vi "Day01-02.vi"() -> ()   [LabVIEW 2021]
uses:
  2b6feea8-4815-4cd8-ae99-f2c110e22a6b.vi
  <vilib>/Comparison/Equal/Equal Functor/Equal Functor.lvclass
panel:
  out "마지막 값":i32
  out "조건적":i32[](array[numeric])
  out "인덱스 하기":i32[](array[numeric])
  out "배열":dbl[](array[numeric])
  out "숫자형 3":dbl
  out "숫자형 2":i32
  in  "STOP 2":bool
  out "x+y 4":dbl
  in  "x 2":dbl
  in  "y 2":dbl
  out "x+y 3":dbl
  in  "y":dbl
  in  "x":dbl
  in  "STOP":bool
  out "숫자형":i32
  out "증가 값":dbl[](array[numeric])
  in  "인덱스":dbl
  in  "원래 값":dbl[](array[numeric])
  out "출력 클러스터 2":cluster{"금액":dbl, "버튼":bool, "상태창":string}
  out "출력 클러스터":cluster{"금액":dbl, "버튼":bool, "상태창":string}
  out "클러스터어어 5":cluster{"숫자랑 배열":dbl[], "버튼":bool, "상태창":string}
  in  "클러스터어어 4":cluster{"숫자랑 배열":dbl[], "버튼":bool, "상태창":string}
  in  "클러스터어어 3":cluster{"금액":dbl, "버튼":bool, "상태창":string}
  in  "클러스터어어 2":cluster{"금액":dbl, "버튼":bool, "상태창":string}
  out "상태창":string
  out "버튼":bool
  out "금액":dbl
  in  "클러스터어어":cluster{"금액":dbl, "버튼":bool, "상태창":string}
  out "연결된 문자열":string
  out "길이":i32[](array[numeric])
  out "x .and. y? 2":bool[](array[boolean])
  out "x .and. y?":bool[](array[boolean])
  out "x+y 2":i32[](array[numeric])
  out "x+y":i32[](array[numeric])
  out "index of element":i32 caption="원소의 인덱스"
  out "추가된 배열 5":dbl[](array[numeric])
  out "추가된 배열 4":dbl[][](array[numeric])
  out "추가된 배열 3":dbl[](array[numeric])
  out "추가된 배열 2":dbl[](array[numeric])
  out "추가된 배열":dbl[](array[numeric])
  # "숫자형 함수의 다형성"
  # "불리언 함수의 다형성"
  # "문자형 함수의 다형성"
  # "문자형 함수의 다형성 2"
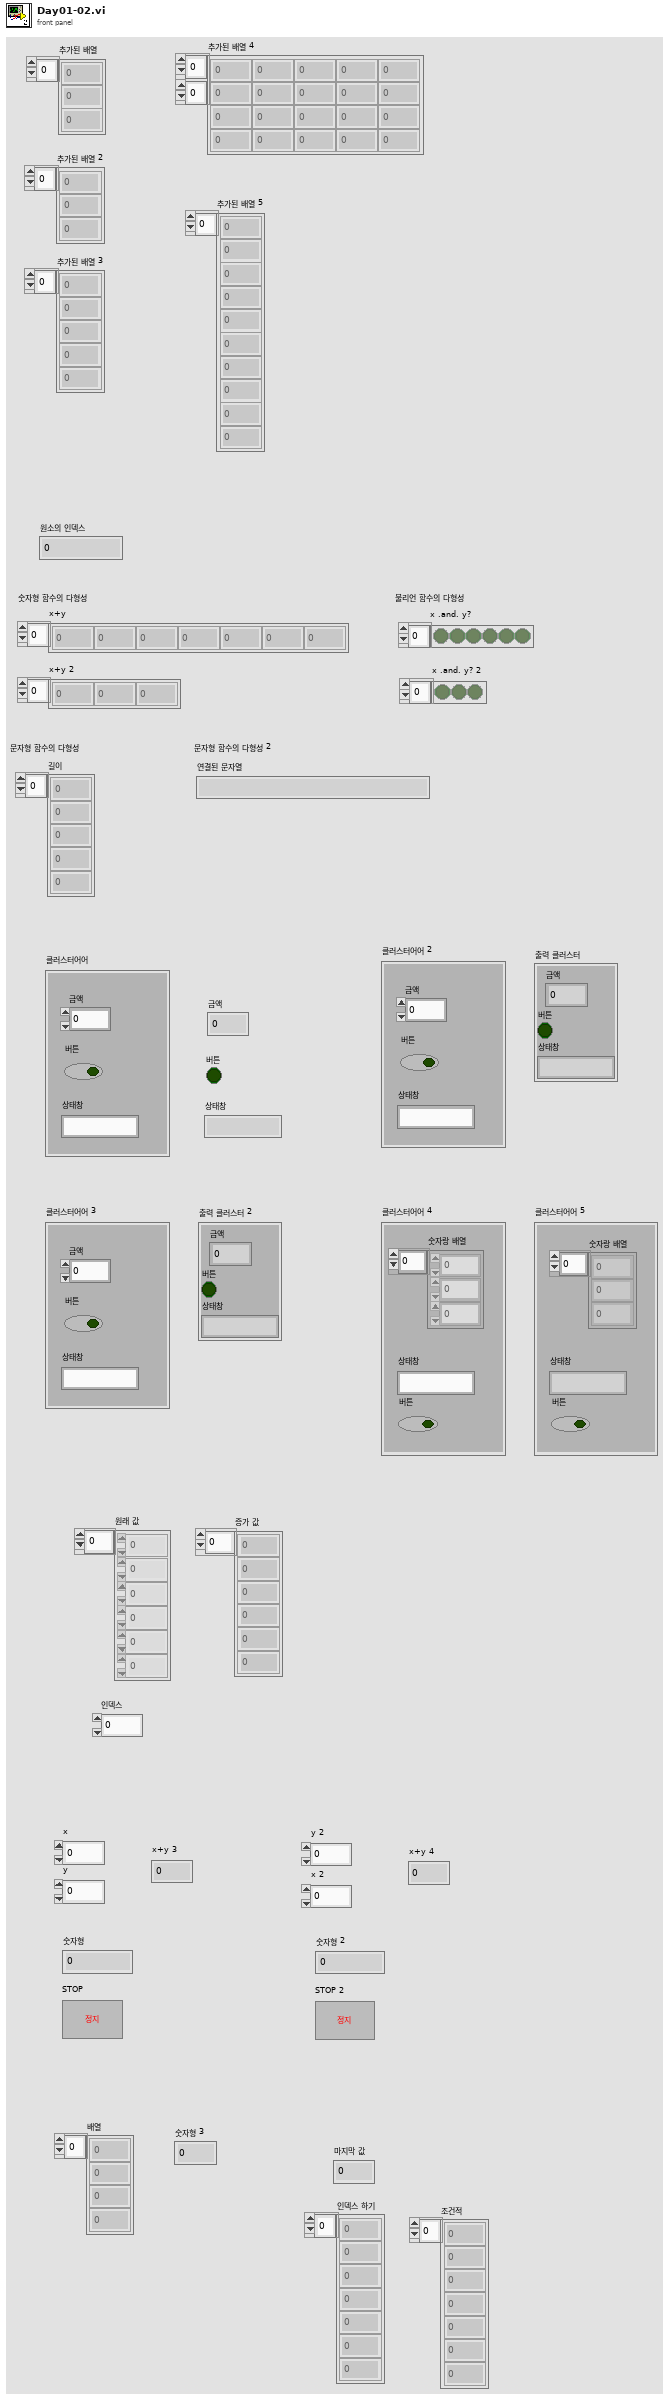
[diagram p1: front panel]
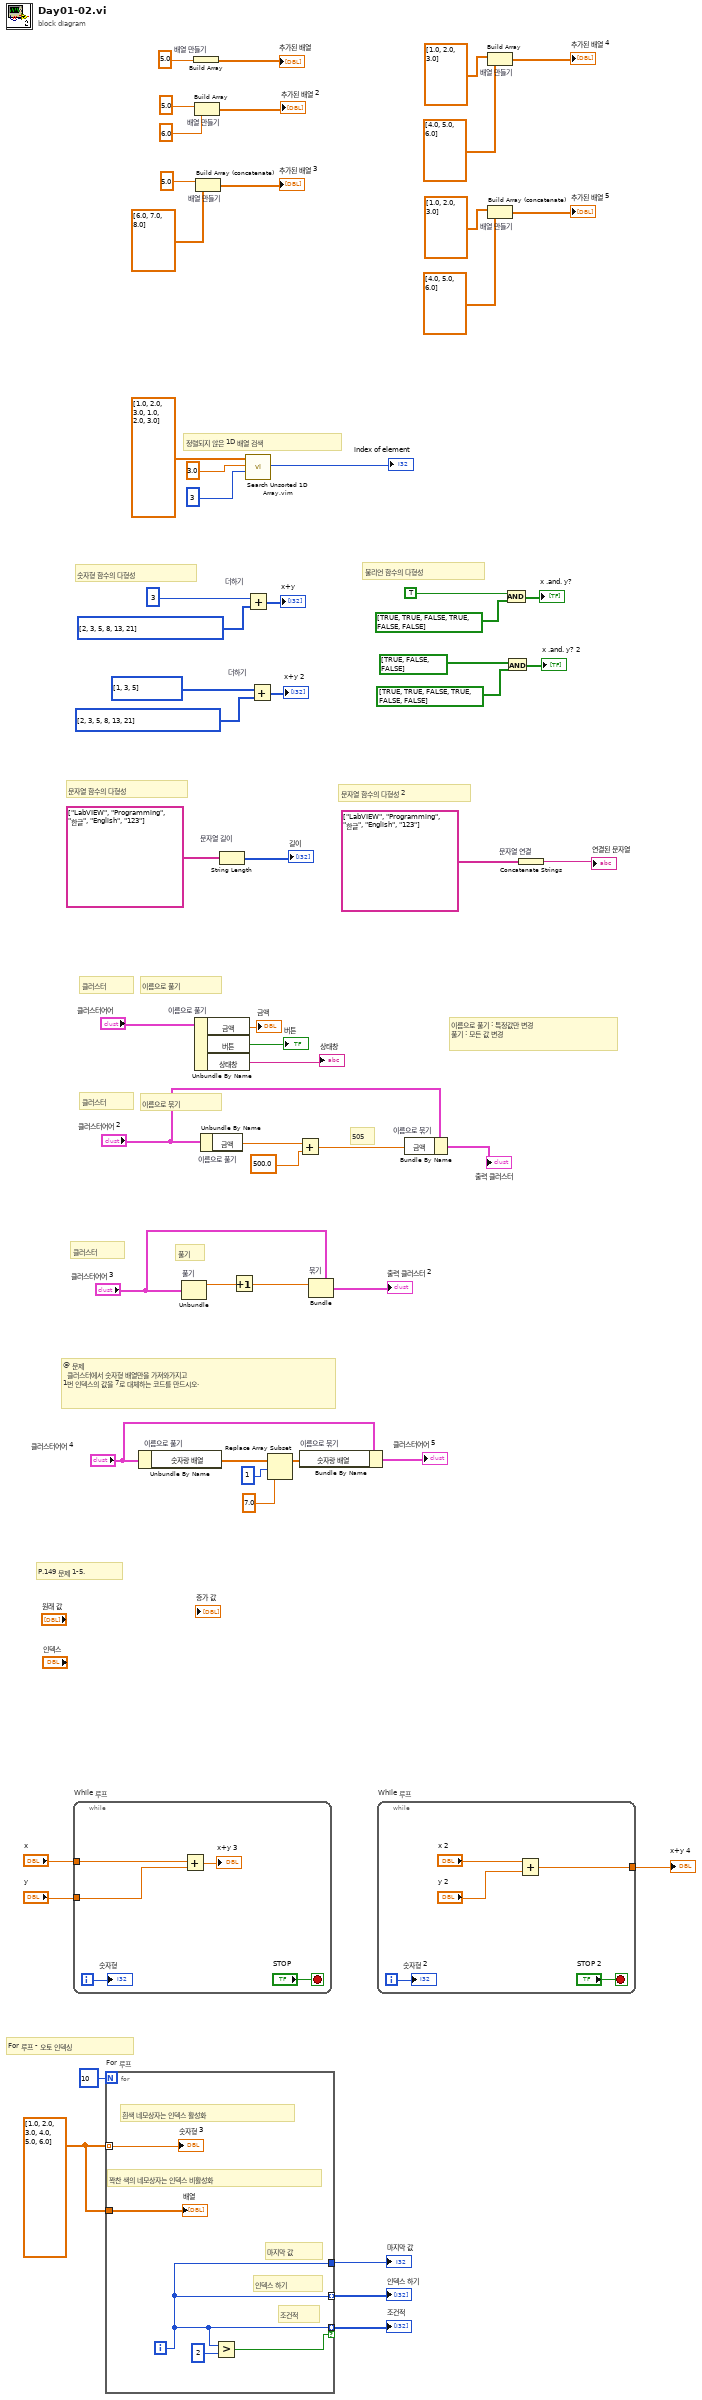
[diagram p0: block diagram]
diagram:
  w4 = dbl[] [1.0, 2.0, 3.0, 4.0, 5.0, 6.0]
  # "For 루프 - 오토 인덱싱"
  # "P.149 문제 1-5."
  # "이름으로 묶기"
  # "505"
  # "@ 문제\n  클러스터에서 숫자형 배열만을 가져와가지고\n1번 인덱스의 값을 7로 대체하는 코드를 만드시오."
  # "클러스터"
  # "이름으로 풀기 : 특정값만 변경\n풀기 : 모든 값 변경"
  # "풀기"
  # "이름으로 풀기"
  # "클러스터"
  # "클러스터"
  # "문자열 함수의 다형성 2"
  # "문자열 함수의 다형성"
  # "불리언 함수의 다형성"
  # "숫자형 함수의 다형성"
  # "정렬되지 않은 1D 배열 검색"
  n1 = while "While 루프" {
    tunnel: "x" -> [w64]
    tunnel: "y" -> [w63]
    i -> [w66]
    stop <- "STOP" stop-if-true
    n2 = Add(x=w64, y=w63) -> (x+y=→"x+y 3":dbl)
    "숫자형" <- w66
  }
  n3 = for "For 루프" {
    N: 10 -> [_]
    tunnel: w4 -> [w71] mode=indexing
    tunnel: w4 -> [w70]
    tunnel: [w69] -> w1
    tunnel: [w69] -> w3 mode=indexing
    tunnel: [w69] -> w2 mode=indexing if=w67
    i -> [w69]
    # "조건적"
    # "인덱스 하기"
    # "마지막 값"
    # "꽉찬 색의 네모상자는 인덱스 비활성화"
    # "흰색 네모상자는 인덱스 활성화"
    n4 = Greater?(x=w69, y=2) -> (0:w67:bool)
    "숫자형 3" <- w71
    "배열" <- w70
  }
  "인덱스 하기" <- w3
  "조건적" <- w2
  "마지막 값" <- w1
  n5 = Unbundle By Name "이름으로 풀기"("클러스터어어 4") -> ("숫자랑 배열"=w18:dbl[])
  n6 = Unbundle "풀기"("클러스터어어 3") -> ("금액"=w23:dbl)  [unwired: 2 out]
  n7 = Build Array "배열 만들기"(5.0 ("원소")) -> (→"추가된 배열":dbl[])
  n8 = Build Array "배열 만들기"(5.0 ("원소"), 6.0 ("원소")) -> (→"추가된 배열 2":dbl[])
  n9 = Unbundle By Name "이름으로 풀기"("클러스터어어") -> ("금액"=→"금액":dbl, "버튼"=→"버튼":bool, "상태창"=→"상태창":string)
  n10 = Build Array (concatenate) "배열 만들기"(5.0 ("원소"), dbl[] [6.0, 7.0, 8.0] ("원소")) -> (→"추가된 배열 3":dbl[])
  n11 = Unbundle By Name "이름으로 풀기"("클러스터어어 2") -> ("금액"=w21:dbl)
  n12 = String Length "문자열 길이"(string=string[] ["LabVIEW", "Programming", "한글", "English", "123"]) -> (length=→"길이":i32[])
  n13 = Increment(x=w23) -> (x+1=w12:dbl)
  n14 = call "Search Unsorted 1D Array.vim"("start index (0)"=3, "element"=3.0, "unsorted 1D array"=dbl[] [1.0, 2.0, 3.0, 1.0, 2.0, 3.0]) -> ("index of element"=→"index of element":i32)  [unwired: 8 in]
  n15 = Add "더하기"(x=3, y=i32[] [2, 3, 5, 8, 13, 21]) -> (x+y=→"x+y":i32[])
  n16 = Add "더하기"(x=i32[] [1, 3, 5], y=i32[] [2, 3, 5, 8, 13, 21]) -> (x+y=→"x+y 2":i32[])
  n17 = Replace Array Subset(array=w18, new element=7.0 ("새 원소/부분배열"), index=1 ("인덱스")) -> (w15:dbl[])
  n18 = Add(x=w21, y=500.0) -> (x+y=w22:dbl)
  n19 = Bundle By Name "이름으로 묶기"(cluster="클러스터어어 4", "숫자랑 배열"=w15) -> (→"클러스터어어 5":cluster{"숫자랑 배열":dbl[], "버튼":bool, "상태창":string})
  n20 = Bundle "묶기"(cluster="클러스터어어 3", "금액"=w12) -> (→"출력 클러스터 2":cluster{"금액":dbl, "버튼":bool, "상태창":string})  [unwired: 2 in]
  n21 = while "While 루프" {
    tunnel: [w72] -> w6
    i -> [w76]
    stop <- "STOP 2" stop-if-true
    n22 = Add(x="x 2", y="y 2") -> (x+y=w72:dbl)
    "숫자형 2" <- w76
  }
  "x+y 4" <- w6
  n23 = Bundle By Name "이름으로 묶기"(cluster="클러스터어어 2", "금액"=w22) -> (→"출력 클러스터":cluster{"금액":dbl, "버튼":bool, "상태창":string})
  n24 = Build Array "배열 만들기"(dbl[] [1.0, 2.0, 3.0] ("원소"), dbl[] [4.0, 5.0, 6.0] ("원소")) -> (→"추가된 배열 4":dbl[][])
  n25 = Build Array (concatenate) "배열 만들기"(dbl[] [1.0, 2.0, 3.0] ("원소"), dbl[] [4.0, 5.0, 6.0] ("원소")) -> (→"추가된 배열 5":dbl[])
  n26 = And(x=TRUE, y=bool[] [TRUE, TRUE, FALSE, TRUE, FALSE, FALSE]) -> (x .and. y?=→"x .and. y?":bool[])
  n27 = And(x=bool[] [TRUE, FALSE, FALSE], y=bool[] [TRUE, TRUE, FALSE, TRUE, FALSE, FALSE]) -> (x .and. y?=→"x .and. y? 2":bool[])
  n28 = Concatenate Strings "문자열 연결"(string[] ["LabVIEW", "Programming", "한글", "English", "123"]) -> (→"연결된 문자열":string)
